vi "Get Object Size.vi"(8 "error in (no error)":errorcluster, 11 "Channel Runtime in":refnum<class "Runtime.Channel.lvclass">) -> (0 "error out":errorcluster, 2 "size in bytes":u64 format="%d bytes", 3 "Channel Runtime out":refnum<class "Runtime.Channel.lvclass">)   [LabVIEW 2016, in "Data Sharing Framework.Runtime.lvlib" / "Runtime.Channel.lvclass"]
uses:
  Runtime.Channel.lvclass
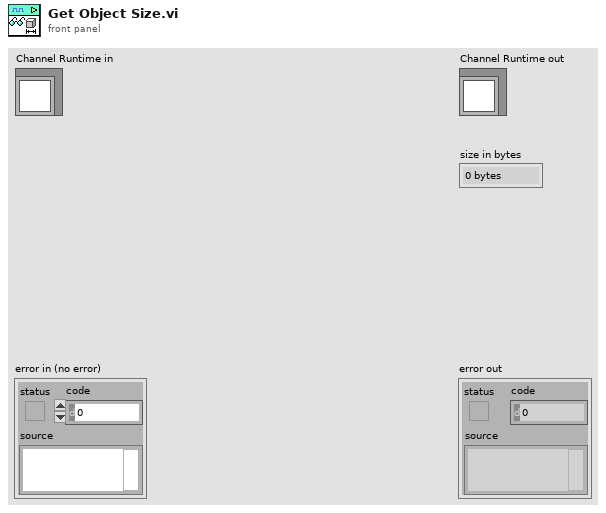
[diagram p1: front panel]
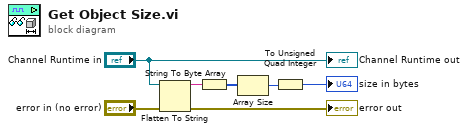
[diagram p0: block diagram]
diagram:
  n1 = Flatten To String(anything="Channel Runtime in", error in (no error)="error in (no error)") -> (data string=w6:string, error out=→"error out":errorcluster)  [unwired: 2 in, 1 out]
  n2 = String To Byte Array(string=w6) -> (unsigned byte array=w7:u8[])
  n3 = Array Size(array=w7) -> (size(s)=w4:i32)
  n4 = To Unsigned Quad Integer(1:w4) -> (0:→"size in bytes":u64)
  "Channel Runtime out" <- "Channel Runtime in"
